vi "Initialize Instrument Engine.vi"(8 "error in (no error)":errorcluster, 9 "Name":string, 11 "Process":refnum<class "Process.lvclass">) -> (0 "error out":errorcluster, 2 "notification":bool, 3 "State Variables":T1)   [LabVIEW 2018, in "Instrument Addon Engine.lvlib"]
uses:
  Instrument Addon Engine.lvlib
  Addon Shared/SubVIs/Constants.vi
  Addon Shared/Instrument Addon Shared.lvlib
  Types/Engine State Variables.ctl
  <vilib>/NI/NIVS Inline Async API/_VS Inline Async API/Process/Process.lvclass
  <vilib>/NI/NIVS Inline Async API/_Data Access Engine/Access Type Classes/ReadWrite/ReadWrite.lvclass
  <vilib>/NI/NIVS Inline Async API/_Data Access Engine/Data Access Engine/Data Access Engine.lvclass
  <vilib>/NI/NIVS Inline Async API/_Data Access Engine/Data Access Engine/Methods/Read.Lookup.vi
  <vilib>/NI/NIVS Inline Async API/_Data Access Engine/Data Access Engine/Methods/Write.Lookup.vi
  <vilib>/NI/NI VeriStand Addon Network Comm/Engine/VeriStand Comm.lvclass
  <vilib>/NI/NIVS Inline Async API/_Data Access Engine/Access Type Classes/Read/Read.lvclass
  <vilib>/NI/NIVS Inline Async API/_Data Access Engine/Data Access Engine/Types/Read.DVR.ctl
  <vilib>/NI/NIVS Inline Async API/_Data Access Engine/Access Type Classes/Write/Write.lvclass
  <vilib>/NI/NIVS Inline Async API/_Data Access Engine/Data Access Engine/Types/Write.DVR.ctl
  <vilib>/NI/NIVS Inline Async API/_Data Access Engine/Data Access Engine/Types/ReadWrite.DVR.ctl
  <vilib>/NI/NIVS Inline Async API/_Data Access Engine/Data Access Engine/Methods/ReadWrite.Lookup.vi
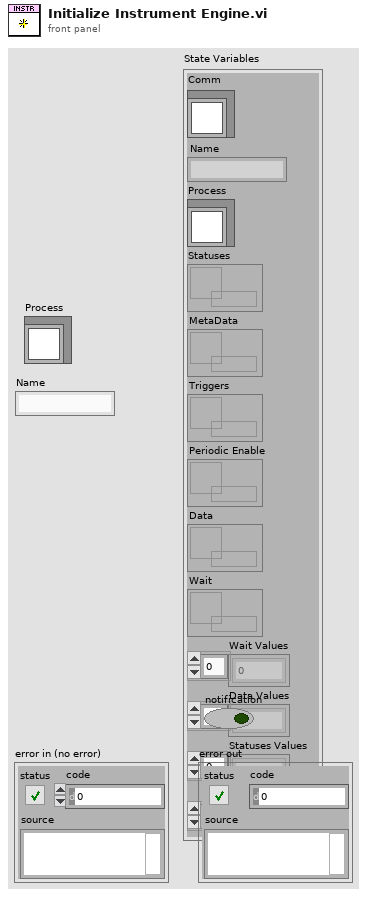
[diagram p1: front panel]
types:
  T1 = typedef "Instrument Addon Engine.lvlib/Engine State Variables.ctl" = cluster{"Comm":refnum<class "VeriStand Comm.lvclass">, "Name":string, "Process":refnum<class "Process.lvclass">, "Statuses":T2, "MetaData":T3, "Triggers":T4, "Periodic Enable":T3, "Data":T2, "Wait":T3, "Wait Values":dbl[], "Data Values":dbl[], "Statuses Values":dbl[], "MetaData Values":dbl[]}
  T2 = typedef "Data Access Engine.lvlib/Data Access Engine.lvclass/Write.DVR.ctl" = refnum<data-value>
  T3 = typedef "Data Access Engine.lvlib/Data Access Engine.lvclass/Read.DVR.ctl" = refnum<data-value>
  T4 = typedef "Data Access Engine.lvlib/Data Access Engine.lvclass/ReadWrite.DVR.ctl" = refnum<data-value>
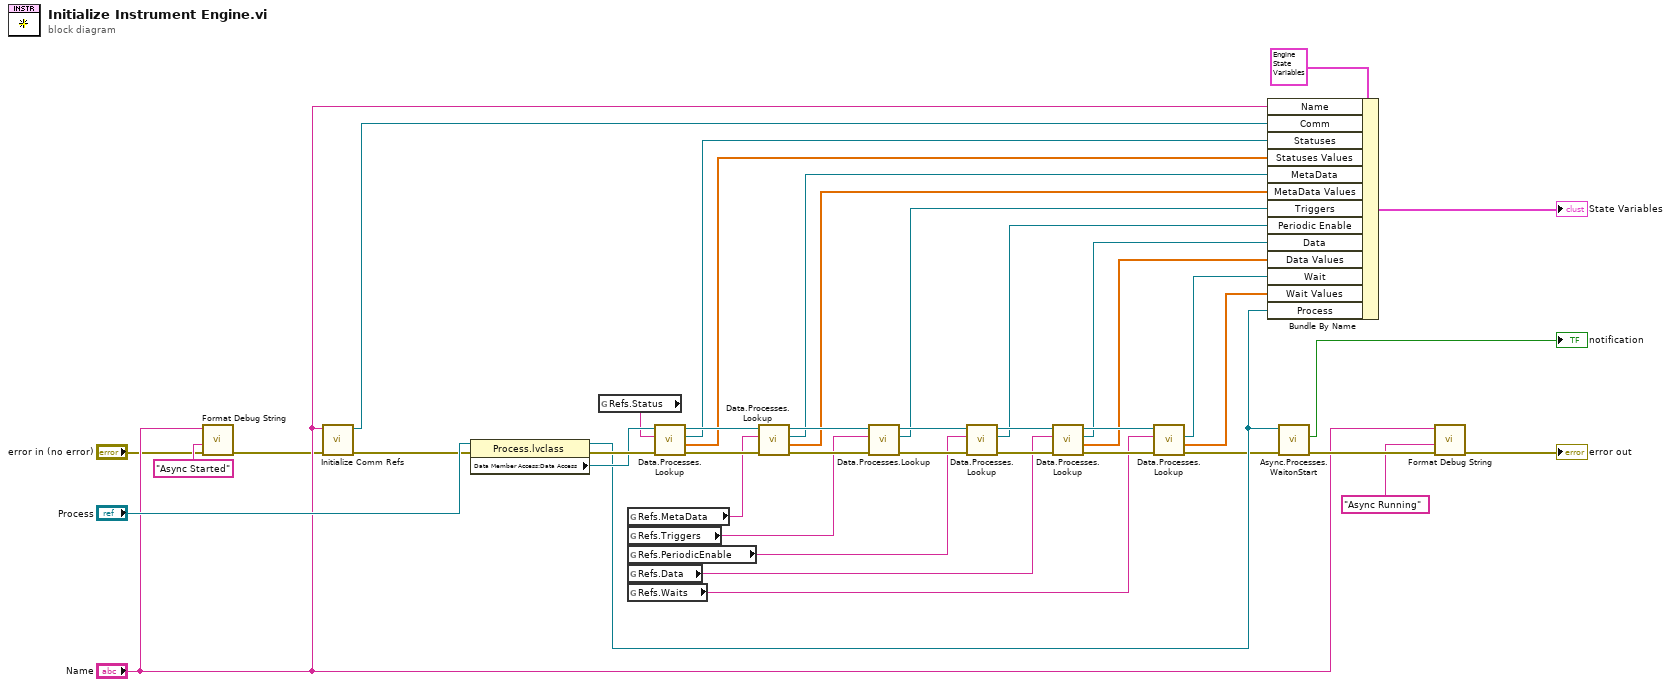
[diagram p0: block diagram]
diagram:
  n1 = call "Format Debug String.vi"("error in (no error)"="error in (no error)", "State"="Async Started" ("string"), "Name"="Name") -> ("error out"=w1:errorcluster)  [unwired: 8 in]
  n2 = call <vilib>:"Initialize Comm Refs.vi"("error in (no error)"=w1, "Name"="Name") -> ("error out"=w9:errorcluster, "Comm.lvclass"=w42:refnum<class "VeriStand Comm.lvclass">)  [unwired: 8 in]
  n3 = property class="Process.lvclass"(reference="Process", error in=w9) -> (reference out=w31:refnum<class "Process.lvclass">, error out=w39:errorcluster, "Data Member Access:Data Access"=w38:refnum<class "Data Access Engine.lvclass">)
  n4 = global read "Constants.vi" "Refs.Status"() -> (w20:string)
  n5 = global read "Constants.vi" "Refs.MetaData"() -> (w19:string)
  n6 = global read "Constants.vi" "Refs.Triggers"() -> (w17:string)
  n7 = global read "Constants.vi" "Refs.PeriodicEnable"() -> (w16:string)
  n8 = global read "Constants.vi" "Refs.Data"() -> (w15:string)
  n9 = global read "Constants.vi" "Refs.Waits"() -> (w14:string)
  n10 = call-poly <vilib>:"Data.Processes.Lookup.vi"("error in (no error)"=w39, "Name"=w20, "Data Access API in"=w38) -> ("error out"=w21:errorcluster, "Initial Values"=w11:dbl[], "Ref"=w8:T2, "Data Access API out"=w37:refnum<class "Data Access Engine.lvclass">)  [unwired: 5 in]
  n11 = call-poly <vilib>:"Data.Processes.Lookup.vi"("error in (no error)"=w21, "Name"=w19, "Data Access API in"=w37) -> ("error out"=w18:errorcluster, "Initial Values"=w12:dbl[], "Ref"=w22:T3, "Data Access API out"=w36:refnum<class "Data Access Engine.lvclass">)  [unwired: 5 in]
  n12 = call-poly <vilib>:"Data.Processes.Lookup.vi"("error in (no error)"=w18, "Name"=w17, "Data Access API in"=w36) -> ("error out"=w24:errorcluster, "Ref"=w23:T4, "Data Access API out"=w35:refnum<class "Data Access Engine.lvclass">)  [unwired: 5 in, 1 out]
  n13 = call-poly <vilib>:"Data.Processes.Lookup.vi"("error in (no error)"=w24, "Name"=w16, "Data Access API in"=w35) -> ("error out"=w25:errorcluster, "Ref"=w26:T3, "Data Access API out"=w34:refnum<class "Data Access Engine.lvclass">)  [unwired: 5 in, 1 out]
  n14 = call-poly <vilib>:"Data.Processes.Lookup.vi"("error in (no error)"=w25, "Name"=w15, "Data Access API in"=w34) -> ("error out"=w27:errorcluster, "Initial Values"=w10:dbl[], "Ref"=w28:T2, "Data Access API out"=w33:refnum<class "Data Access Engine.lvclass">)  [unwired: 5 in]
  n15 = call-poly <vilib>:"Data.Processes.Lookup.vi"("error in (no error)"=w27, "Name"=w14, "Data Access API in"=w33) -> ("error out"=w30:errorcluster, "Initial Values"=w13:dbl[], "Ref"=w29:T3)  [unwired: 5 in, 1 out]
  n16 = Bundle By Name(cluster=T1 {"Comm"=refnum, "Name"="", "Process"=refnum, "Statuses"=refnum, "MetaData"=refnum, "Triggers"=refnum, "Periodic Enable"=refnum, "Data"=refnum, "Wait"=refnum, "Wait Values"=[], "Data Values"=[], "Statuses Values"=[], "MetaData Values"=[]} ("State Variables"), "Name"="Name", "Comm"=w42, "Statuses"=w8, "Statuses Values"=w11, "MetaData"=w22, "MetaData Values"=w12, "Triggers"=w23, "Periodic Enable"=w26, "Data"=w28, "Data Values"=w10, "Wait"=w29, "Wait Values"=w13, "Process"=w31) -> (→"State Variables":T1)
  n17 = call <vilib>:"Async.Processes.WaitonStart.vi"("error in (no error)"=w30, "Process"=w31) -> ("error out"=w6:errorcluster, "Execute"=→"notification":bool)  [unwired: 7 in, 1 out]
  n18 = call "Format Debug String.vi"("error in (no error)"=w6, "State"="Async Running" ("string"), "Name"="Name") -> ("error out"=→"error out":errorcluster)  [unwired: 8 in]
